vi "Set Hardware Configuration File.vi"(8 "error in":errorcluster, 10 "hardware configuration file path":path, 11 "Ballard MIL-STD 1553 custom device in":T1 format="%.0x") -> (0 "error out":errorcluster, 3 "Ballard MIL-STD 1553 custom device out":T1 format="%.0x")   [LabVIEW 2020, in "Ballard MIL-STD-1553 Scripting.lvlib"]
doc: "Specifies the <b>hardware configuration file path</b>. The hardware configuration file is deployed to the RT target and must be consistent with the system configuration for successful deployment and avionics bus communication."
uses:
  Ballard MIL-STD-1553 Scripting.lvlib
  <vilib>/NI VeriStand/Custom Device API/Custom Device Item Ref.ctl
  <vilib>/NI VeriStand/Custom Device API/Dependent File Optional Info.ctl
  Constants.vi
  <vilib>/NI VeriStand/Custom Device API/Set Item Property (Dependent File).vi
  <vilib>/NI VeriStand/Custom Device API/Custom Device API.lvlib
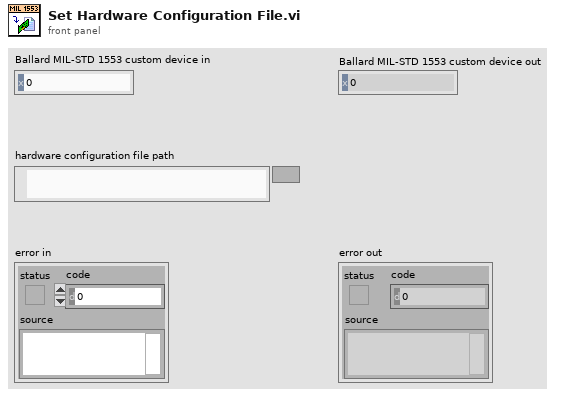
[diagram p1: front panel]
types:
  T1 = typedef "Custom Device API.lvlib/Custom Device Item Ref.ctl" = u64
  T2 = typedef "Custom Device API.lvlib/Dependent File Optional Info.ctl" = cluster{"Version":string, "RTDestination":path, "ForceDownload":bool, "SupportedTarget":string, "MD5":string}
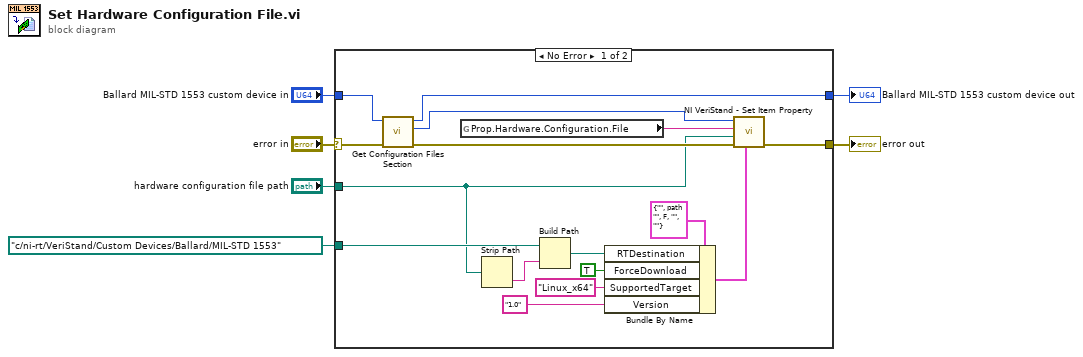
[diagram p0: block diagram]
diagram:
  n1 = case shown="No Error" "error in" {
    selector: "error in" -> [w13 w24]
    tunnel: "Ballard MIL-STD 1553 custom device in" -> [w11 w23]
    tunnel: [w22 w24] -> w5
    tunnel: [w10 w23] -> w3
    tunnel: "hardware configuration file path" -> [w8 _]
    tunnel: path "c:/ni-rt/VeriStand/Custom Devices/Ballard/MIL-STD 1553" ("RTDestination") -> [w18 _]
    frame No Error {
      n2 = call "Get Configuration Files Section.vi"("error in"=w13, "custom device in"=w11) -> ("error out"=w12:errorcluster, "configuration files section"=w7:T1, "custom device out"=w10:T1)  [unwired: 7 in]
      n3 = global read "Constants.vi" "Prop.Hardware.Configuration.File"() -> (w9:string)
      n4 = Strip Path(path=w8) -> (name=w19:string)  [unwired: 1 out]
      n5 = Build Path(base path=w18, name or relative path=w19) -> (appended path=w17:path)
      n6 = Bundle By Name(cluster=T2 {"Version"="", "RTDestination"=path "", "ForceDownload"=FALSE, "SupportedTarget"="", "MD5"=""} ("OptionalInfo"), "RTDestination"=w17, "ForceDownload"=TRUE, "SupportedTarget"="Linux_x64", "Version"="1.0") -> (w20:T2)
      n7 = call-poly <vilib>:"NI VeriStand - Set Item Property.vi"("OptionalInfo"=w20, "error in (no error)"=w12, "Path"=w8, "Property Name"=w9, "Item Ref in"=w7) -> ("error out"=w22:errorcluster)  [unwired: 4 in, 2 out]
    }
    frame Error {
    }
  }
  "error out" <- w5
  "Ballard MIL-STD 1553 custom device out" <- w3
